vi "New Queue Logger.vi"(8 "error in (no error)":errorcluster, 9 "log queue (new)":refnum<queue>) -> (0 "error out":errorcluster, 1 "log queue (out)":refnum<queue>, 3 "WebSocket Queue Logger out":refnum<class "WebSocket Queue Logger.lvclass">)   [LabVIEW 2019, in "WebSocket Server Toolkit.lvlib" / "WebSocket Queue Logger.lvclass"]
uses:
  WebSocket Queue Logger.lvclass
  WebSocket Queue Logger.lvclass/WebSocket Queue Logger.ctl
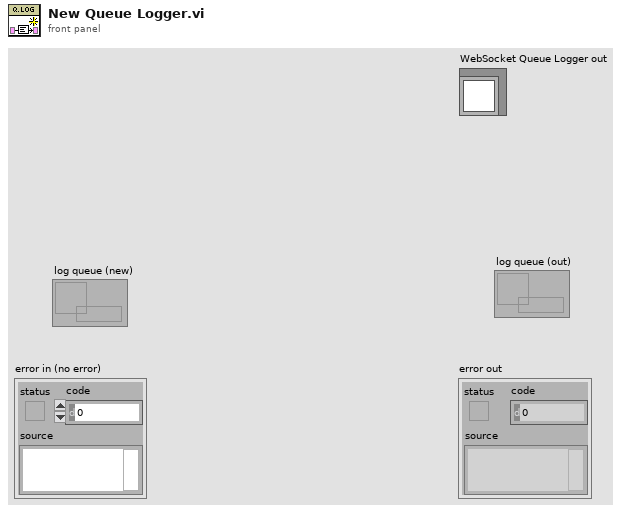
[diagram p1: front panel]
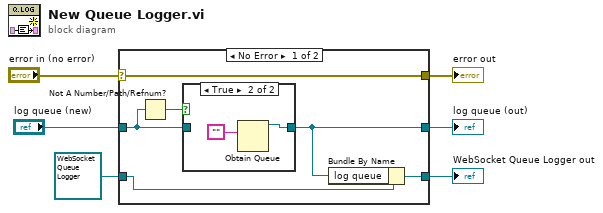
[diagram p0: block diagram]
diagram:
  n1 = case shown="No Error" "error in (no error)" {
    selector: "error in (no error)" -> [w11 w18]
    tunnel: [w11 w18] -> w5
    tunnel: [w10 w17] -> w3
    tunnel: refnum<class "WebSocket Queue Logger.lvclass"> refnum ("WebSocket Queue Logger in") -> [w12 w17]
    tunnel: [w9 w16] -> w2
    tunnel: "log queue (new)" -> [w7 w16]
    frame No Error {
      n2 = Not A Number/Path/Refnum?(number/path/refnum=w7) -> (NaN/Path/Refnum?=w8:bool)
      n3 = case shown="True" w8 {
        tunnel: [w13 w14] -> w9
        tunnel: w7 -> [w13 _]
        frame False {
        }
        frame True {
          n4 = Obtain Queue(element data type="") -> (queue out=w14:refnum<queue>)  [unwired: 4 in, 2 out]
        }
      }
      n5 = Bundle By Name(cluster=w12, "log queue"=w9) -> (w10:refnum<class "WebSocket Queue Logger.lvclass">)
    }
    frame Error {
    }
  }
  "error out" <- w5
  "WebSocket Queue Logger out" <- w3
  "log queue (out)" <- w2
